vi "HapticSTM.vi"() -> ()   [LabVIEW 2019]
uses:
  SubVIs/GlobalClicksHeight.vi
  <userlib>/HapticSTM/HapticSTM.lvlib
panel:
  out "Safetip":bool
  out "Forces":cluster{"Fy":dbl, "Fz":dbl, "Fx":dbl} {"Fy" format="%.1f"; "Fz" format="%.1f"; "Fx" format="%.1f"}
  out "Position":cluster{"X":dbl, "Y":dbl, "Z pen":dbl, "Z":dbl}
  out "Frame Properties":cluster{"Ox":dbl, "Oy":dbl, "Fw":dbl, "Fh":dbl}
  in  "Save":bool
  in  "# Sample Points":i32=4096
  in  "Depth (pA)":dbl=280.0
  in  "Shift (in)":dbl format="%.1f"
  in  "Hardness":dbl=0.7 format="%.1f"
  in  "Scaling?":u16(ring) items=["Medium", "Large", "Small"]
  out "Setpoint (pA)":dbl
  in  "Maximum (pA)":dbl=7000.0
  out "Filtered Current (pA)":dbl format="%.1f"
  out "Current (pA)":dbl format="%.1f"
  out "Z Write":dbl format="%^.1e"
  in  "Planing?":bool
  in  "Mode":u16(ring) items=["Log w/ Exp Z", "Log w/ Lin Z", "Coulomb Force", "Lennard Jones", "r^6"]
  in  "Reset Clicks":bool
  out "Clicks":i32
  in  "STOP":bool
  in  "START":bool
  # "Super Ultra Mega Haptic STM Controller 3000"
  # "Haptic Pen"
  # "Nanonis"
  # "Position"
  # "Z Controller"
  # "Force"
  # "Frame"
  # "Surface"
  # "Options"
  # "Current"
  # "No"
  # "Yes"
  # "Planing"
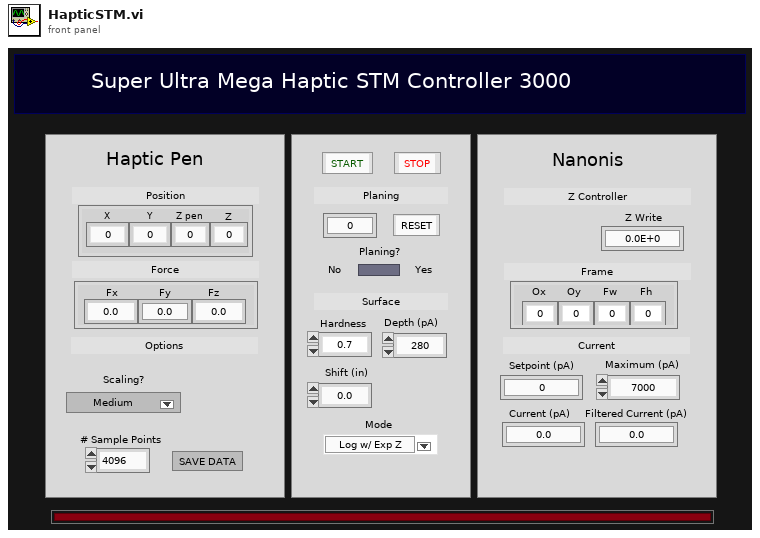
[diagram p1: front panel]
types:
  T1 = cluster{"X Origin (nm)":dbl, "Y Origin (nm)":dbl, "FW (nm)":dbl, "FH (nm)":dbl}
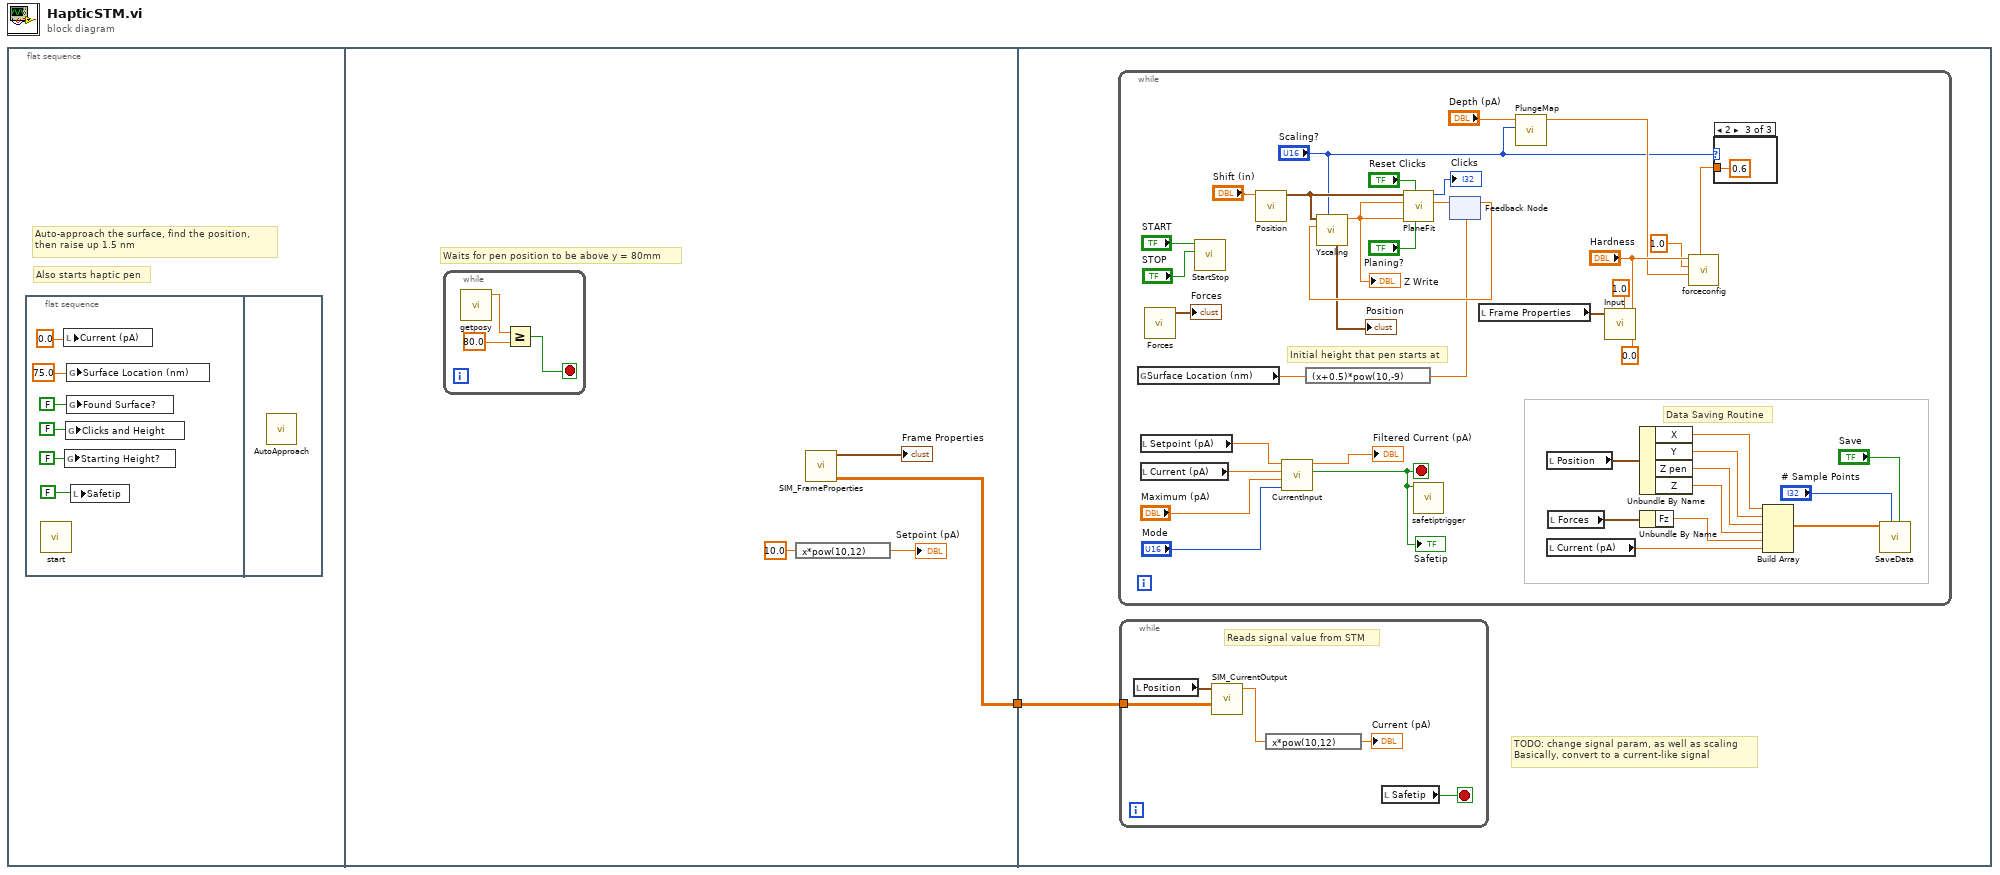
[diagram p0: block diagram]
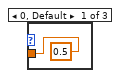
[diagram p2: hidden frame]
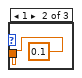
[diagram p3: hidden frame]
diagram:
  n1 = flat-sequence {
    tunnel: [w8] -> w1
    tunnel: w1 -> [w15]
    frame #0 {
      # "Also starts haptic pen"
      # "Auto-approach the surface, find the position, \nthen raise up 1.5 nm"
      n2 = flat-sequence {
        frame #0 {
          n3 = call <userlib>:"start.vi"() -> ()  [unwired: 11 in, 1 out]
          n4 = local write "Current (pA)"(0.0 ("Current (pA)")) -> ()
          n5 = global write "GlobalClicksHeight.vi" "Starting Height?"(FALSE ("Clicks and Height")) -> ()
          n6 = global write "GlobalClicksHeight.vi" "Clicks and Height"(FALSE ("Clicks and Height")) -> ()
          n7 = global write "GlobalClicksHeight.vi" "Surface Location (nm)"(75.0 ("Surface Location")) -> ()
          n8 = global write "GlobalClicksHeight.vi" "Found Surface?"(FALSE ("Clicks and Height")) -> ()
          n9 = local write "Safetip"(FALSE ("Safe Tip?")) -> ()
        }
        frame #1 {
          n10 = call "AutoApproach.vi"() -> ()  [unwired: 12 in]
        }
      }
    }
    frame #1 {
      # "Waits for pen position to be above y = 80mm"
      n11 = while {
        stop <- w12 stop-if-true
        n12 = call <userlib>:"getposy.vi"() -> ("function return"=w14:dbl)  [unwired: 11 in]
        n13 = Greater Or Equal?(x=w14, y=80.0) -> (x >= y?=w12:bool)
      }
      n14 = expression code="x*pow(10,12)"(sgl 10.0 ("Z Controller setpoint")) -> (→"Setpoint (pA)":sgl)
      n15 = call "SIM_FrameProperties.vi"() -> ("data"=w8:dbl[][], "Frame Properties"=→"Frame Properties":T1)  [unwired: 10 in]
    }
    frame #2 {
      # "TODO: change signal param, as well as scaling\nBasically, convert to a current-like signal"
      n16 = while {
        stop <- w21 stop-if-true
        # "Data Saving Routine"
        # "Initial height that pen starts at"
        n17 = global read "GlobalClicksHeight.vi" "Surface Location (nm)"() -> (w32:dbl)
        n18 = local read "Setpoint (pA)"() -> (w30:dbl)
        n19 = local read "Current (pA)"() -> (w29:dbl)
        n20 = call "Forces.vi"() -> ("Forces"=→"Forces":cluster{"Fy":dbl, "Fz":dbl, "Fx":dbl})  [unwired: 11 in]
        n21 = call "StartStop.vi"("STOP"="STOP", "START"="START") -> ()  [unwired: 10 in]
        n22 = call "Position.vi"("Shift"="Shift (in)") -> ("Position"=w39:cluster{"X":dbl, "Y":dbl, "Zpen":dbl})  [unwired: 10 in]
        n23 = call "CurrentInput.vi"("Mode"="Mode", "Maximum (pA)"="Maximum (pA)", "Current (pA)"=w29, "Setpoint (pA)"=w30) -> ("Safetip?"=w21:bool, "Filtered Current (pA)"=→"Filtered Current (pA)":dbl)  [unwired: 6 in]
        "Safetip" <- w21
        n24 = expression code="(x+0.5)*pow(10,-9)"(w32) -> (w31:dbl)
        n25 = call <userlib>:"safetiptrigger.vi"("triggered"=w21) -> ()  [unwired: 11 in]
        n26 = feedback #1(w31) -> (w41:dbl)
        n27 = call "Yscaling.vi"("Scaling?"="Scaling?", "Plane Height (m)"=w41, 11:w39) -> ("y scaled (m)"=w28:dbl, "Position"=→"Position":cluster{"X":dbl, "Y":dbl, "Z pen":dbl, "Z":dbl})  [unwired: 6 in, 1 out]
        "Z Write" <- w28
        n28 = call "PlaneFit.vi"("Planing y/n?"="Planing?", "Reset Clicks"="Reset Clicks", "Y PEN"=w28, "Nano Z"=w28, "Position"=w39) -> ("Plane Height (m)"=w54:dbl, "Clicks"=→"Clicks":i32)  [unwired: 4 in, 1 out]
        n29 = feedback-in #1(w54) -> ()
        n30 = local read "Frame Properties"() -> (w40:cluster{"Ox":dbl, "Oy":dbl, "Fw":dbl, "Fh":dbl})
        n31 = call "PlungeMap.vi"("Scaling?"="Scaling?", "Input (pA)"="Depth (pA)") -> ("output"=w27:dbl)  [unwired: 9 in]
        n32 = local read "Position"() -> (w37:cluster{"X":dbl, "Y":dbl, "Z pen":dbl, "Z":dbl})
        n33 = local read "Current (pA)"() -> (w23:dbl)
        n34 = local read "Forces"() -> (w25:cluster{"Fy":dbl, "Fz":dbl, "Fx":dbl})
        n35 = call "Input.vi"("Current * 10^input"=0.0, "Sensitivity"="Hardness", "Drag"=1.0, "Frame Properties (Remapped)"=w40) -> ()  [unwired: 6 in, 2 out]
        n36 = Unbundle By Name(w37) -> ("X"=w36:dbl, "Y"=w35:dbl, "Z pen"=w34:dbl, "Z"=w33:dbl)
        n37 = Unbundle By Name(w25) -> ("Fz"=w24:dbl)
        n38 = case shown="2" "Scaling?" {
          tunnel: [0.5 0.1 0.6] -> w44
          frame 0, Default {
          }
          frame 1 {
          }
          frame 2 {
          }
        }
        n39 = call <userlib>:"forceconfig.vi"("spc"=w44, "c"=w27, "b"=1.0, "a"="Hardness") -> ()  [unwired: 8 in]
        n40 = Build Array(w36, w35, w34, w33, w24, w23) -> (w60:dbl[])
        n41 = call "SaveData.vi"("Save"="Save", "# Sample Points"="# Sample Points", "Data"=w60) -> ()  [unwired: 9 in]
      }
      n42 = while {
        tunnel: w15 -> [w16]
        stop <- w19 stop-if-true
        # "Reads signal value from STM"
        n43 = local read "Position"() -> (w18:cluster{"X":dbl, "Y":dbl, "Z pen":dbl, "Z":dbl})
        n44 = call "SIM_CurrentOutput.vi"("array"=w16, "Position 2"=w18) -> ("Current Out (pA)"=w17:dbl)  [unwired: 8 in, 1 out]
        n45 = expression code="x*pow(10,12)"(w17) -> (→"Current (pA)":dbl)
        n46 = local read "Safetip"() -> (w19:bool)
      }
    }
  }
